vi "zoom.vi"(8 "error in (no error)":errorcluster, 10 "zoom factor":dbl=1.0, 11 "GenericTrajectory in":refnum<class "TrajectoryDL091126GenericVoxel.lvclass">) -> (0 "error out":errorcluster, 3 "GenericTrajectory out":refnum<class "TrajectoryDL091126GenericVoxel.lvclass">)   [LabVIEW 2010, in "TrajectoryDL091126GenericVoxel.lvclass"]
uses:
  TrajectoryDL091126GenericVoxel.lvclass
  common/enumerations/x_y_z_enumeration.ctl
  common/enumerations/functional_global_action_enum.ctl
  TrajectoryDL091126GenericVoxel.lvclass/TrajectoryDL091126GenericVoxel.ctl
  common/classes/ErrorController/ErrorController/class_data.vi
  common/classes/ErrorController/ErrorController/ErrorController.lvclass
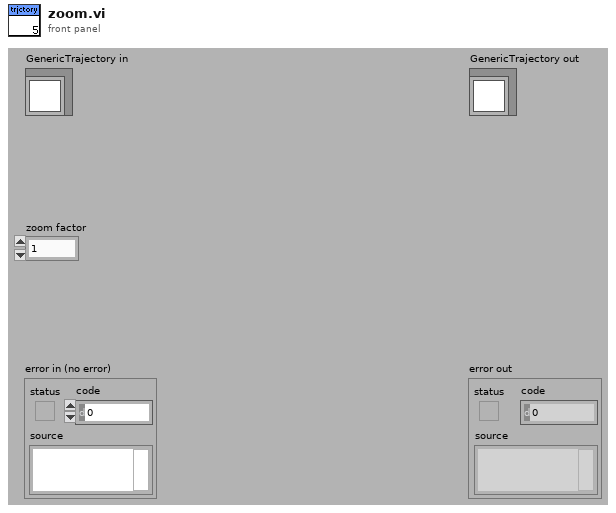
[diagram p1: front panel]
types:
  T1 = typedef "x_y_z_enumeration.ctl" = enum16{"x", "y", "z"}
  T2 = typedef "functional_global_action_enum.ctl" = enum16{"get", "set", "reset"}
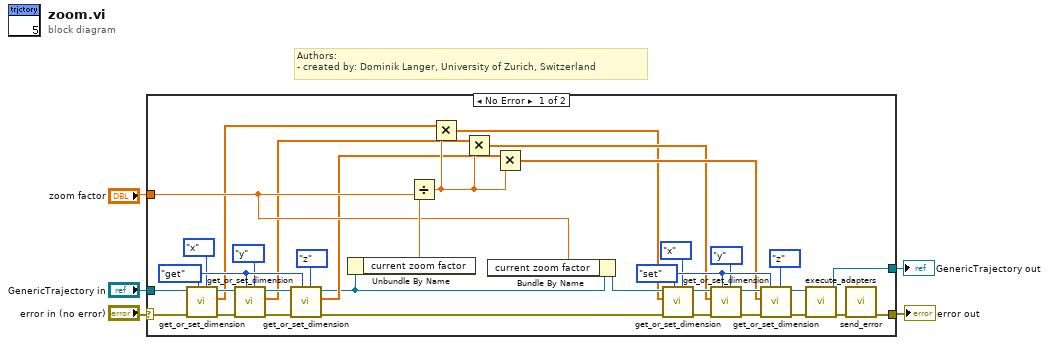
[diagram p0: block diagram]
diagram:
  # "Authors: \n- created by: Dominik Langer, University of Zurich, Switzerland"
  n1 = case shown="No Error" "error in (no error)" {
    selector: "error in (no error)" -> [w31 w42]
    tunnel: [w6 w42] -> w4
    tunnel: [w37 w41] -> w2
    tunnel: "GenericTrajectory in" -> [w30 w41]
    tunnel: "zoom factor" -> [w39 _]
    frame No Error {
      w22 = functional_global_action_enum."set" ("action")
      w36 = functional_global_action_enum."get" ("action")
      n2 = call-dynamic "get_or_set_dimension.vi"("dimension"=x_y_z_enumeration."x", "action"=w36, "error in (no error)"=w31, "GenericTrajectory in"=w30) -> ("error out"=w33:errorcluster, "pixel values out (single dimension)"=w29:dbl[unit][], "GenericTrajectory out"=w34:refnum<class "TrajectoryDL091126GenericVoxel.lvclass">)  [unwired: 2 in, 3 out]
      n3 = call-dynamic "get_or_set_dimension.vi"("dimension"=x_y_z_enumeration."y", "action"=w36, "error in (no error)"=w33, "GenericTrajectory in"=w34) -> ("error out"=w32:errorcluster, "pixel values out (single dimension)"=w28:dbl[unit][], "GenericTrajectory out"=w35:refnum<class "TrajectoryDL091126GenericVoxel.lvclass">)  [unwired: 2 in, 3 out]
      n4 = call-dynamic "get_or_set_dimension.vi"("dimension"=x_y_z_enumeration."z", "action"=w36, "error in (no error)"=w32, "GenericTrajectory in"=w35) -> ("error out"=w21:errorcluster, "pixel values out (single dimension)"=w27:dbl[unit][], "GenericTrajectory out"=w18:refnum<class "TrajectoryDL091126GenericVoxel.lvclass">)  [unwired: 2 in, 3 out]
      n5 = Unbundle By Name(w18) -> ("current zoom factor"=w40:dbl)
      n6 = Divide(x=w40, y=w39) -> (x/y=w38:dbl)
      n7 = Multiply(x=w29, y=w38) -> (x*y=w14:dbl[unit][])
      n8 = Multiply(x=w28, y=w38) -> (x*y=w15:dbl[unit][])
      n9 = Bundle By Name(cluster=w18, "current zoom factor"=w39) -> (w17:refnum<class "TrajectoryDL091126GenericVoxel.lvclass">)
      n10 = Multiply(x=w27, y=w38) -> (x*y=w16:dbl[unit][])
      n11 = call-dynamic "get_or_set_dimension.vi"("dimension"=x_y_z_enumeration."x", "action"=w22, "error in (no error)"=w21, "pixel values in (single dimension)"=w14, "GenericTrajectory in"=w17) -> ("error out"=w25:errorcluster, "GenericTrajectory out"=w24:refnum<class "TrajectoryDL091126GenericVoxel.lvclass">)  [unwired: 1 in, 4 out]
      n12 = call-dynamic "get_or_set_dimension.vi"("dimension"=x_y_z_enumeration."y", "action"=w22, "error in (no error)"=w25, "pixel values in (single dimension)"=w15, "GenericTrajectory in"=w24) -> ("error out"=w26:errorcluster, "GenericTrajectory out"=w23:refnum<class "TrajectoryDL091126GenericVoxel.lvclass">)  [unwired: 1 in, 4 out]
      n13 = call-dynamic "get_or_set_dimension.vi"("dimension"=x_y_z_enumeration."z", "action"=w22, "error in (no error)"=w26, "pixel values in (single dimension)"=w16, "GenericTrajectory in"=w23) -> ("error out"=w20:errorcluster, "GenericTrajectory out"=w19:refnum<class "TrajectoryDL091126GenericVoxel.lvclass">)  [unwired: 1 in, 4 out]
      n14 = call-dynamic "execute_adapters.vi"("error in (no error)"=w20, "GenericTrajectory in"=w19) -> ("error out"=w7:errorcluster, "GenericTrajectory out"=w37:refnum<class "TrajectoryDL091126GenericVoxel.lvclass">)  [unwired: 8 out]
      n15 = call "send_error.vi"("error in (no error)"=w7) -> ("error out"=w6:errorcluster)  [unwired: 10 in]
    }
    frame Error {
    }
  }
  "error out" <- w4
  "GenericTrajectory out" <- w2
